vi "Billard2023.vi"() -> ()   [LabVIEW 2023]
panel:
  in  "Marker Style":string
  in  "Border Loss Color":u32(colorbox)
  out "Image sequence":picture
  out "error out":errorcluster
  out "Standard error":string
  in  "Border Hit Style":string
  in  "Line Style":string
  in  "Border Win Color":u32(colorbox)
  in  "Create Score Sheet":bool
  in  "Folder Path":path
  # "Billiard 2023"
  # "Choose one of the following line styles:\n[   -   --   -.   :   ]"
  # "Choose one of the following border hit styles:\n[   o   +   *   .   x   square   diamond   ]"
  # "Choose one of the following marker styles:\n[   .   +   *   x   square   ]"
  # "Choose the border win color"
  # "Choose the border loss color"
  # "Roy Turk 34 55 73\nSelim Sherif 34 60 35"
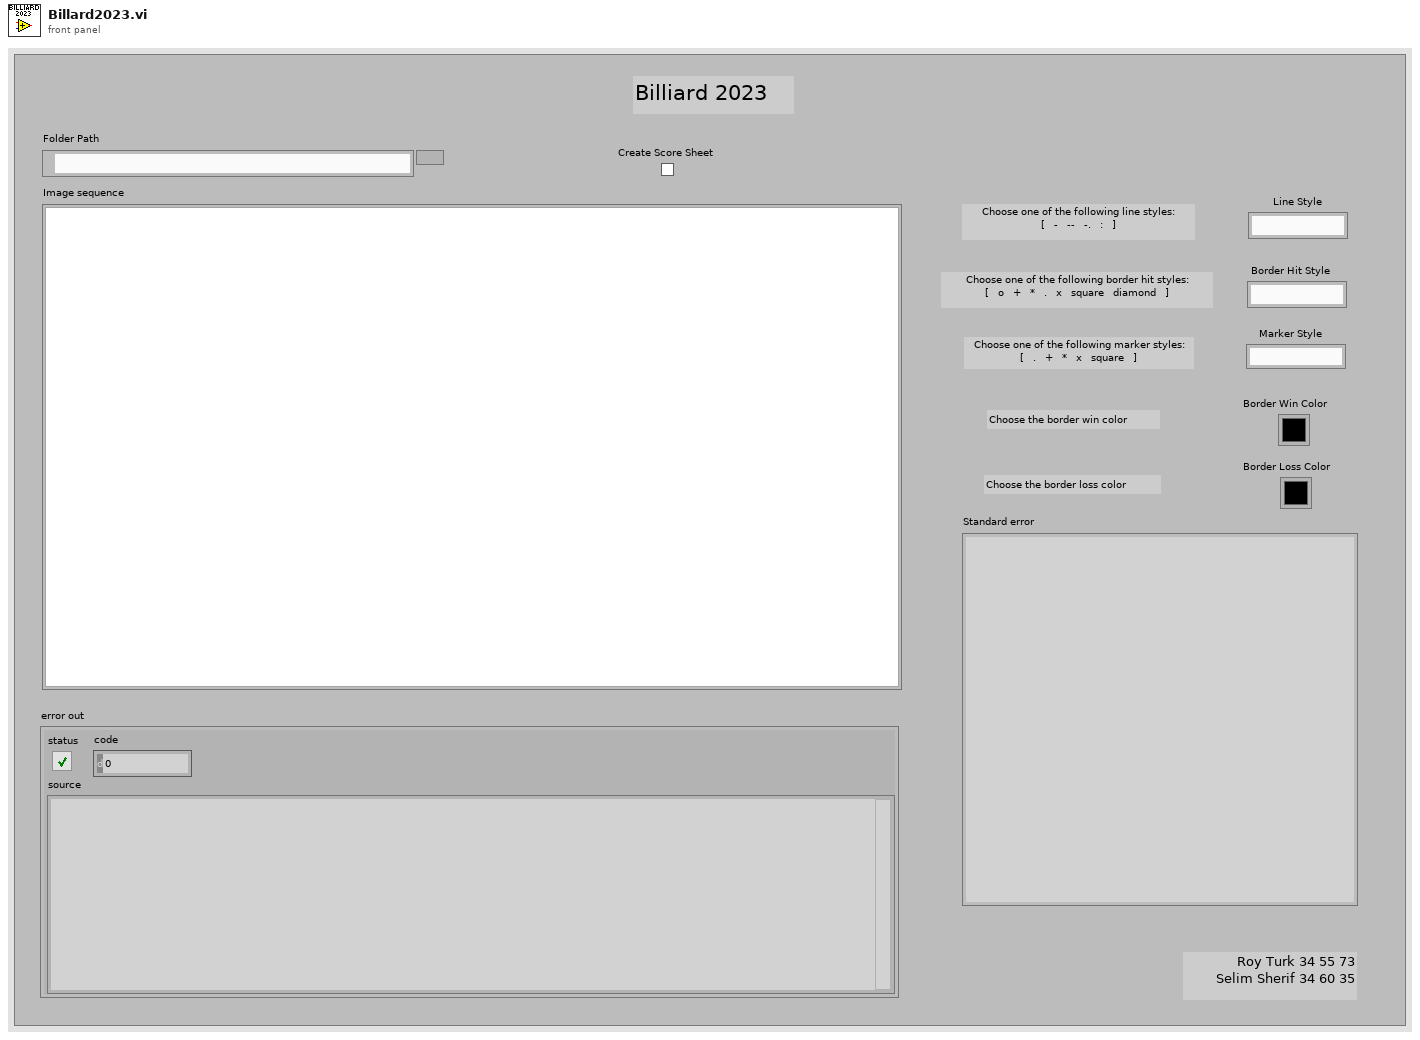
[diagram p1: front panel]
types:
  T1 = cluster{"Lmin":i32, "Lmax":i32, "Cmin":i32, "Cmax":i32}
  T2 = cluster{"Red_X":i32, "Red_Y":i32, "Red_S":i32, " Yellow_X":i32, "Yellow_Y":i32, "Yellow_S":i32, "White_X":i32, "White_Y":i32, "White_S":i32}
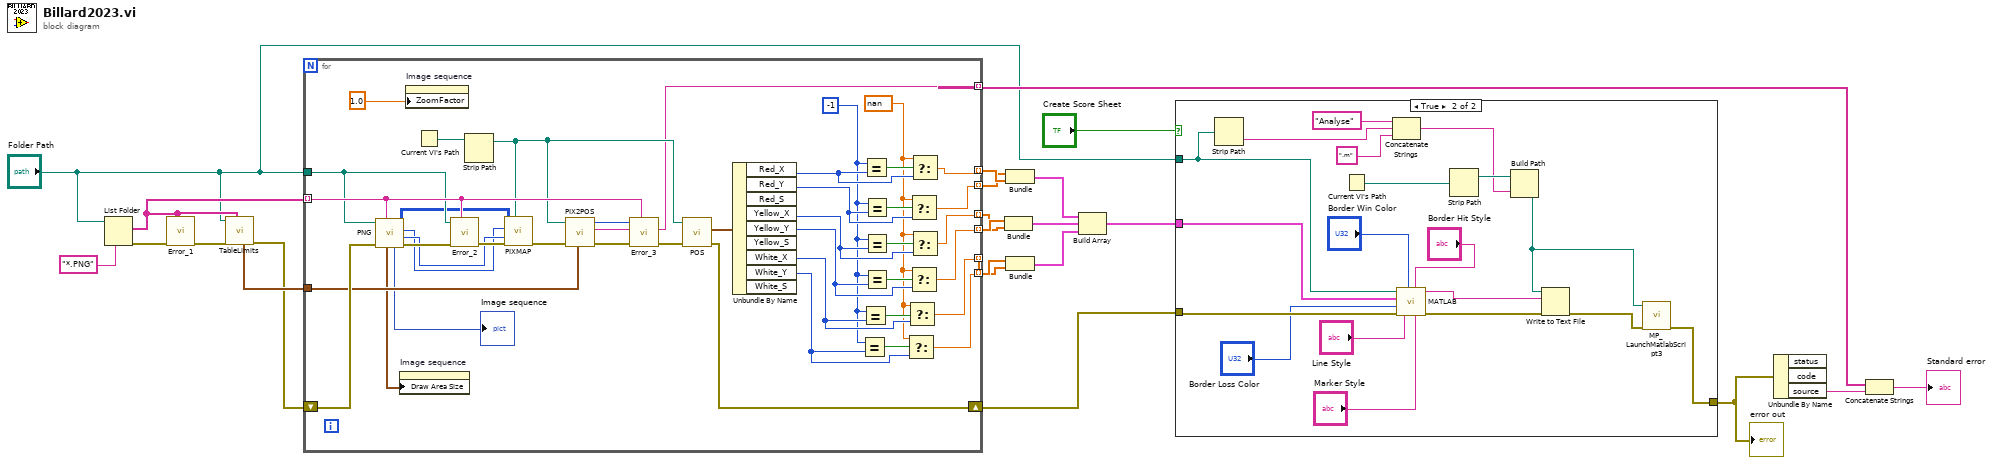
[diagram p0: block diagram]
diagram:
  n1 = List Folder(path="Folder Path", pattern="*.PNG") -> (filenames=w19:string[], error out=w22:errorcluster)  [unwired: 2 in, 2 out]
  n2 = call "Error_1.vi"("PNGs in folder"=w19, "error in (no error)"=w22) -> ("error out"=w21:errorcluster)  [unwired: 9 in]
  n3 = call "TableLimits.vi"("PNGs in folder"=w19, "error in (no error)"=w21, "Folder path"="Folder Path") -> ("error out"=w2:errorcluster, "Table limits"=w20:T1)  [unwired: 7 in]
  n4 = for {
    shift-right: [w48] -> w17
    shift-left: w2 -> [w65]
    tunnel: w20 -> [w47]
    tunnel: "Folder Path" -> [w56]
    tunnel: w19 -> [w59] mode=indexing
    tunnel: [w50] -> w3 mode=indexing
    tunnel: [w37] -> w16 mode=indexing
    tunnel: [w36] -> w15 mode=indexing
    tunnel: [w35] -> w13 mode=indexing
    tunnel: [w30] -> w14 mode=indexing
    tunnel: [w28] -> w11 mode=indexing
    tunnel: [w24] -> w12 mode=indexing
    w27 = nan
    w26 = -1
    n5 = call "PNG.vi"("Current PNG filename"=w59, "error in (no error)"=w65, "Folder path"=w56) -> ("error out"=w64:errorcluster, "Height"=w55:i16, "Width"=w54:i16, "2D Pixmap"=w53:u32[][], "PNG Picture"=→"Image sequence":picture, "Cluster"=w44:cluster{"Width":dbl, "Height":dbl})  [unwired: 3 in]
    n6 = property on="Image sequence" class="Pict"("Draw Area Size"=w44) -> ()  [unwired: 2 in, 2 out]
    n7 = property on="Image sequence" class="Pict"("ZoomFactor"=1.0) -> ()  [unwired: 2 in, 2 out]
    n8 = Current VI's Path() -> (path=w52:path)
    n9 = call "Error_2.vi"("Current PNG Filename"=w59, "error in (no error)"=w64, "Folder Path"=w56) -> ("error out"=w63:errorcluster)  [unwired: 8 in]
    n10 = Strip Path(path=w52) -> (stripped path=w51:path)  [unwired: 1 out]
    n11 = call "PIXMAP.vi"("IV Folder Path"=w51, "error in (no error)"=w63, "Height"=w55, "Width"=w54, "2D Pixmap"=w53) -> ("error out"=w62:errorcluster)  [unwired: 6 in]
    n12 = call "PIX2POS.vi"("Table limits"=w47, "error in (no error)"=w62, "VI Folder Path"=w51) -> ("error out"=w61:errorcluster, "C std err"=w58:string, "C return"=w57:i32)  [unwired: 6 in]
    n13 = call "Error_3.vi"("Current PNG filename"=w59, "error in (no error)"=w61, "Standard error"=w58, "C return"=w57) -> ("error out"=w60:errorcluster, "Standard error"=w50:string)  [unwired: 6 in]
    n14 = call "POS.vi"("error in (no error)"=w60, "VI Folder Path"=w51) -> ("error out"=w48:errorcluster, "Balls"=w49:T2)  [unwired: 7 in, 1 out]
    n15 = Unbundle By Name(w49) -> ("Red_X"=w42:i32, "Red_Y"=w40:i32, "Yellow_X"=w38:i32, "Yellow_Y"=w33:i32, "White_X"=w31:i32, "White_Y"=w25:i32)  [unwired: 3 out]
    n16 = Equal?(x=w26, y=w25) -> (x = y?=w29:bool)
    n17 = Equal?(x=w26, y=w31) -> (x = y?=w32:bool)
    n18 = Equal?(x=w26, y=w42) -> (x = y?=w43:bool)
    n19 = Equal?(x=w26, y=w40) -> (x = y?=w41:bool)
    n20 = Equal?(x=w26, y=w38) -> (x = y?=w39:bool)
    n21 = Equal?(x=w26, y=w33) -> (x = y?=w34:bool)
    n22 = Select(t=w27, s=w29, f=w25) -> (s? t:f=w24:dbl)
    n23 = Select(t=w27, s=w32, f=w31) -> (s? t:f=w28:dbl)
    n24 = Select(t=w27, s=w41, f=w40) -> (s? t:f=w36:dbl)
    n25 = Select(t=w27, s=w34, f=w33) -> (s? t:f=w30:dbl)
    n26 = Select(t=w27, s=w43, f=w42) -> (s? t:f=w37:dbl)
    n27 = Select(t=w27, s=w39, f=w38) -> (s? t:f=w35:dbl)
  }
  n28 = Bundle(w14, w13) -> (w9:cluster{dbl[], dbl[]})  [unwired: 1 in]
  n29 = Bundle(w15, w16) -> (w10:cluster{dbl[], dbl[]})  [unwired: 1 in]
  n30 = Bundle(w12, w11) -> (w8:cluster{dbl[], dbl[]})  [unwired: 1 in]
  n31 = Build Array(w10, w9, w8) -> (w7:cluster{dbl[], dbl[]}[])
  n32 = case shown="True" "Create Score Sheet" {
    tunnel: w17 -> [w66 w84]
    tunnel: w7 -> [_ w78]
    tunnel: [w66 w73] -> w6
    tunnel: "Folder Path" -> [_ w70]
    frame False {
    }
    frame True {
      n33 = Strip Path(path=w70) -> (name=w69:string)  [unwired: 1 out]
      n34 = Current VI's Path() -> (path=w72:path)
      n35 = Concatenate Strings("Analyse", w69, ".m") -> (w75:string)
      n36 = call "MATLAB.vi"("Marker Style"="Marker Style", "Border Hit Style"="Border Hit Style", "Line Style"="Line Style", "Border Win Color"="Border Win Color", "error in (no error)"=w84, "Border Loss Color"="Border Loss Color", "Ball Coordinates"=w78, "Folder Path"=w70) -> ("error out"=w80:errorcluster, "MATLAB Script"=w79:string)  [unwired: 2 in]
      n37 = Strip Path(path=w72) -> (stripped path=w85:path)  [unwired: 1 out]
      n38 = Build Path(base path=w85, name or relative path=w75) -> (appended path=w71:path)
      n39 = Write to Text File(file (use dialog)=w71, text=w79, error in=w80) -> (error out=w74:errorcluster)  [unwired: 1 in, 2 out]
      n40 = call "MP_LaunchMatlabScript3.vi"("error in (no error)"=w74, "matlab script with path"=w71) -> ("error out"=w73:errorcluster)  [unwired: 5 in, 4 out]
    }
  }
  "error out" <- w6
  n41 = Unbundle By Name(w6) -> ("source"=w5:string)  [unwired: 2 out]
  n42 = Concatenate Strings(w3, w5) -> (→"Standard error":string)
